vi "Stop Core.vi"(10 "final error code":i32, 11 "Hardware in":refnum<class "Hardware.lvclass">) -> (3 "Hardware out":refnum<class "Hardware.lvclass">)   [LabVIEW 2015, in "Hardware.lvlib" / "Hardware.lvclass"]
doc: "(<B>Filename</B>: Actor Framework.lvlib:Actor.lvclass:Stop Core.vi)\n\nDefines what the actor does before it stops. Use the <B>final error code</B> input to determine whether the actor shut down in response to an error.\n\nBy default, this method does nothing. A descendant class may override it to define behavior, such as shutting down any processes the actor initiated in its override of the Actor Core method."
uses:
  Hardware.lvclass
  <vilib>/ActorFramework/Actor/Actor.lvclass
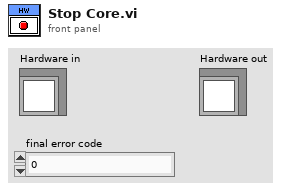
[diagram p1: front panel]
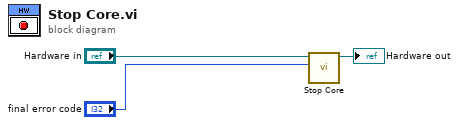
[diagram p0: block diagram]
diagram:
  n1 = call-parent "Stop Core.vi"("final error code"="final error code", "Actor in"="Hardware in") -> ("Actor out"=→"Hardware out":refnum<class "Hardware.lvclass">)  [unwired: 9 in]
